vi "2D_LDA_Time_scale_estimate.vi"(2 "Average Frequency Hz":dbl, 3 "Time":dbl[](array[numeric]), 4 "Velocity 2":dbl[](array[numeric]), 5 "Velocity":dbl[](array[numeric])) -> (0 "Estimated Time Scale BSA2":dbl, 1 "Estimated Time Scale BSA1":dbl)   [LabVIEW 2011]
uses:
  Globals/Meas_global.vi
  <vilib>/Analysis/1siggen.llb/Ramp Pattern by Samples.vi
  <vilib>/Analysis/NI_AALBase.lvlib
  <vilib>/gmath/NI_Gmath.lvlib
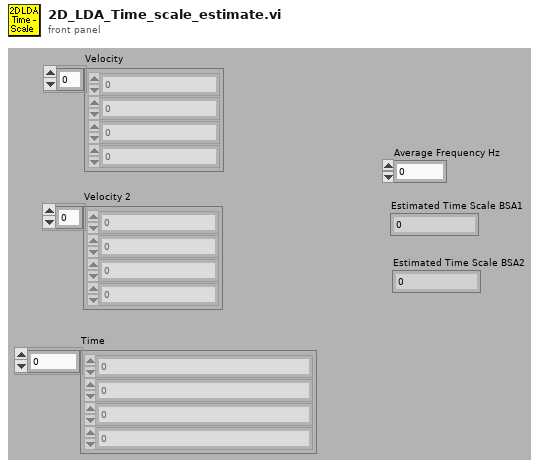
[diagram p1: front panel]
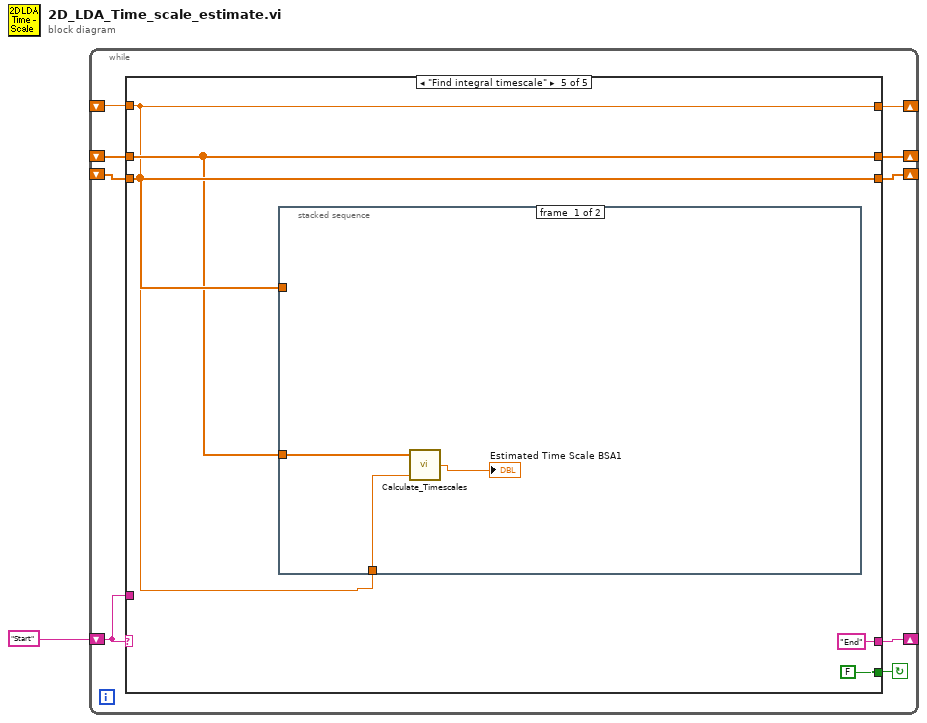
[diagram p0: block diagram]
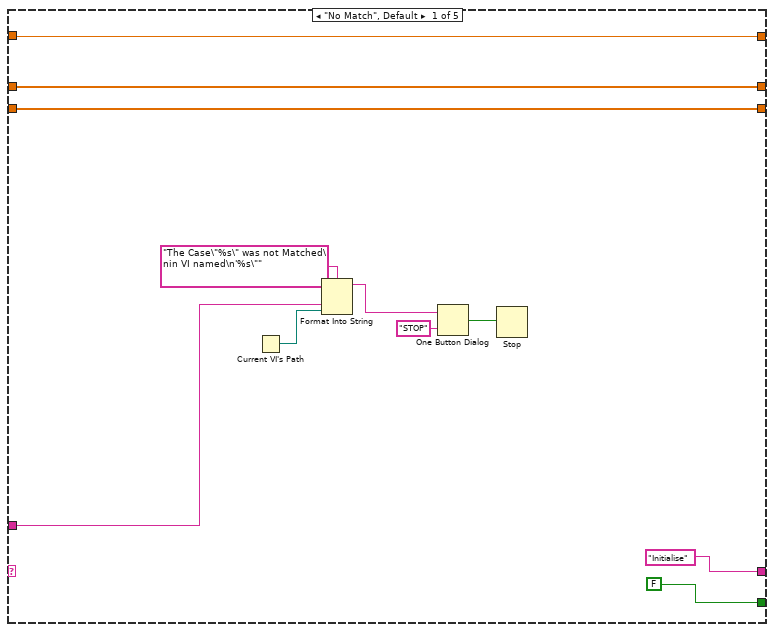
[diagram p2: hidden frame]
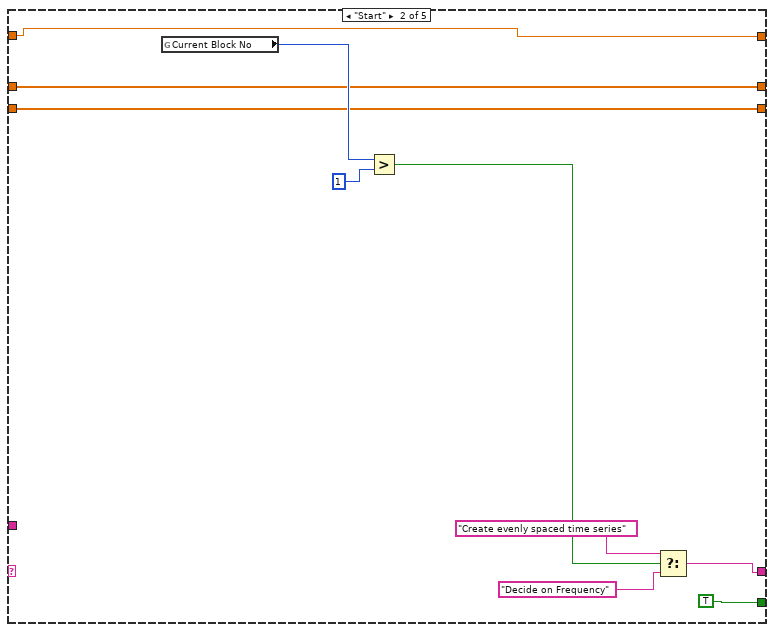
[diagram p3: hidden frame]
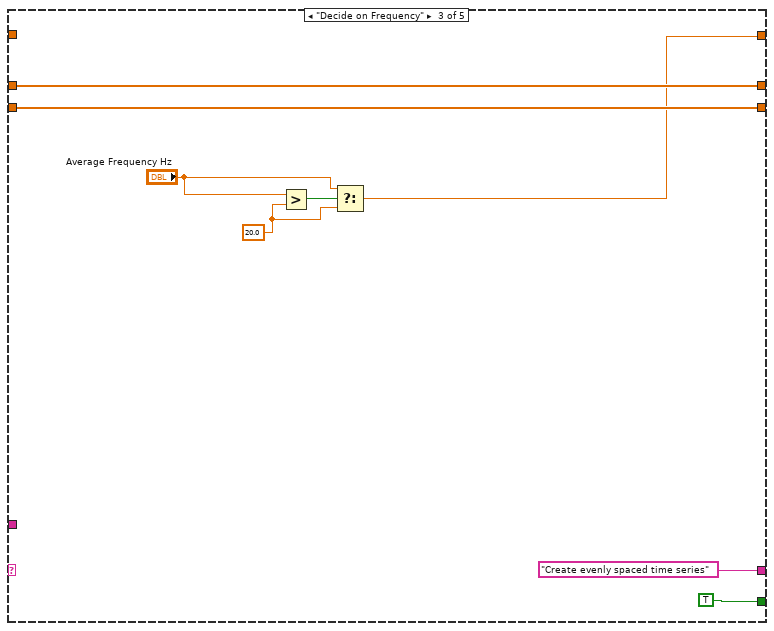
[diagram p4: hidden frame]
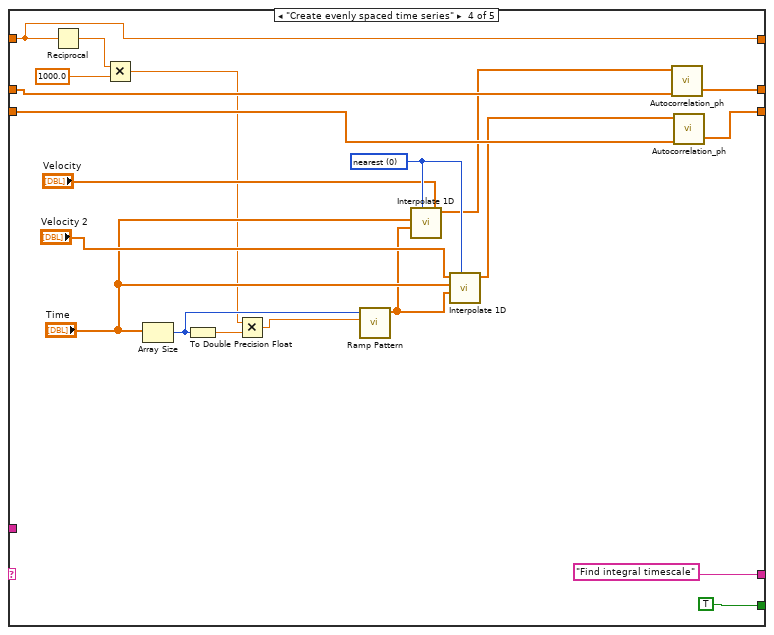
[diagram p5: hidden frame]
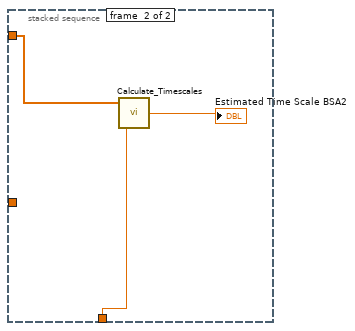
[diagram p6: hidden frame]
diagram:
  n1 = while {
    shift-left: "Start" -> [w8]
    shift-right: [w9] -> _
    shift-right: [w7] -> _
    shift-left: _ -> [w6]
    shift-right: [w5] -> _
    shift-left: _ -> [w4]
    shift-right: [w2] -> _
    shift-left: _ -> [w3]
    stop <- w10 continue-if-true
    n2 = case shown="\"Find integral timescale\"" w8 {
      tunnel: [FALSE TRUE TRUE TRUE FALSE] -> w10
      tunnel: ["Initialise" w30 "Create evenly spaced time series" "Find integral timescale" "End"] -> w9
      tunnel: w8 -> [w16 _ _ _ _]
      tunnel: [w13 w26 w33 w55 w60] -> w7
      tunnel: w6 -> [w13 w26 _ w55 w60]
      tunnel: [w12 w25 w35 w51 w61] -> w5
      tunnel: w4 -> [w12 w25 w35 w54 w61]
      tunnel: w3 -> [w11 w23 w34 w53 w62]
      tunnel: [w11 w23 w34 w52 w62] -> w2
      frame "No Match", Default {
        n3 = Current VI's Path() -> (path=w15:path)
        n4 = Format Into String(format string="The Case\"%s\" was not Matched\nin VI named\n'%s\"" ("Format String"), w16, w15) -> (resulting string=w19:string)  [unwired: 2 in, 1 out]
        n5 = One Button Dialog(message=w19, button name ("OK")="STOP") -> (true=w17:bool)
        n6 = Stop(stop? (T)=w17) -> ()
      }
      frame "Start" {
        n7 = global read "Meas_global.vi" "Current Block No"() -> (w27:i32)
        n8 = Greater?(x=w27, y=1) -> (0:w29:bool)
        n9 = Select(t="Create evenly spaced time series", s=w29, f="Decide on Frequency") -> (s? t:f=w30:string)
      }
      frame "Decide on Frequency" {
        w36 = 20.0 ("y")
        n10 = Greater?(x="Average Frequency Hz", y=w36) -> (0:w37:bool)
        n11 = Select(t="Average Frequency Hz", s=w37, f=w36) -> (s? t:f=w33:dbl)
      }
      frame "Create evenly spaced time series" {
        w46 = 0 items=["nearest", "linear", "spline", "cubic Hermite", "Lagrange"] ("method")
        n12 = Reciprocal(x=w55) -> (1/x=w57:dbl)
        n13 = Multiply(x=w57, y=1000.0) -> (x*y=w40:dbl)
        n14 = Array Size(array="Time") -> (size(s)=w50:i32)
        n15 = To Double Precision Float(number=w50) -> (double precision float=w41:dbl)
        n16 = Multiply(x=w40, y=w41) -> (x*y=w49:dbl)
        n17 = call-poly <vilib>:"Ramp Pattern.vi"("end"=w49, "samples"=w50) -> ("Ramp Pattern"=w44:dbl[])  [unwired: 8 in, 1 out]
        n18 = call <vilib>:"Interpolate 1D.vi"("method"=w46, "xi"=w44, "X"="Time", "Y"="Velocity") -> ("yi"=w42:dbl[])  [unwired: 5 in, 2 out]
        n19 = call <vilib>:"Interpolate 1D.vi"("method"=w46, "xi"=w44, "X"="Time", "Y"="Velocity 2") -> ("yi"=w47:dbl[])  [unwired: 5 in, 2 out]
        n20 = call "Autocorrelation_ph.vi"("X"=w42, "Autocorrelation of X"=w54) -> ("Autocorrelation of X"=w51:dbl[])  [unwired: 3 in, 1 out]
        n21 = call "Autocorrelation_ph.vi"("X"=w47, "Autocorrelation of X"=w53) -> ("Autocorrelation of X"=w52:dbl[])  [unwired: 3 in, 1 out]
      }
      frame "Find integral timescale" {
        n22 = stacked-sequence {
          tunnel: w61 -> [w67 _]
          tunnel: w62 -> [_ w70]
          tunnel: w60 -> [w66 w69]
          frame #0 {
            n23 = call "Calculate_Timescales.vi"("Sampling Frequency (Hz)"=w66, "Autocorrelation"=w67) -> ("Time Scale estimate (s)"=→"Estimated Time Scale BSA1":dbl)  [unwired: 1 in]
          }
          frame #1 {
            n24 = call "Calculate_Timescales.vi"("Sampling Frequency (Hz)"=w69, "Autocorrelation"=w70) -> ("Time Scale estimate (s)"=→"Estimated Time Scale BSA2":dbl)  [unwired: 1 in]
          }
        }
      }
    }
  }
